vi "oef12.vi"() -> ()   [LabVIEW 2021]
panel:
  out "array sum":dbl
  out "result":dbl[][](array[numeric])
  in  "stop":bool
  out "kernel-sum":dbl[][](array[numeric])
  out "result":dbl
  out "inputElement":i8
  out "kernelElement":dbl
  out "rowKernel":i8[](array[numeric])
  out "rowInput":i8[](array[numeric])
  in  "kernel":dbl[][](array[numeric])
  out "Array":i8[][](array[numeric])
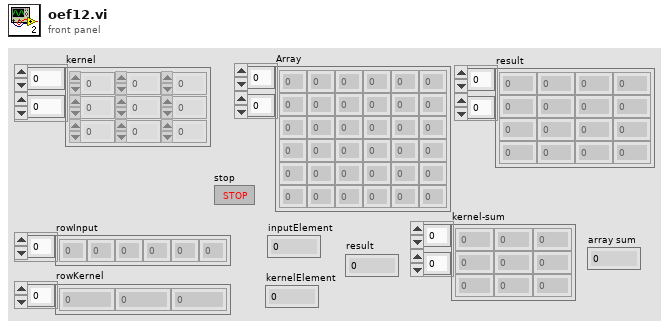
[diagram p1: front panel]
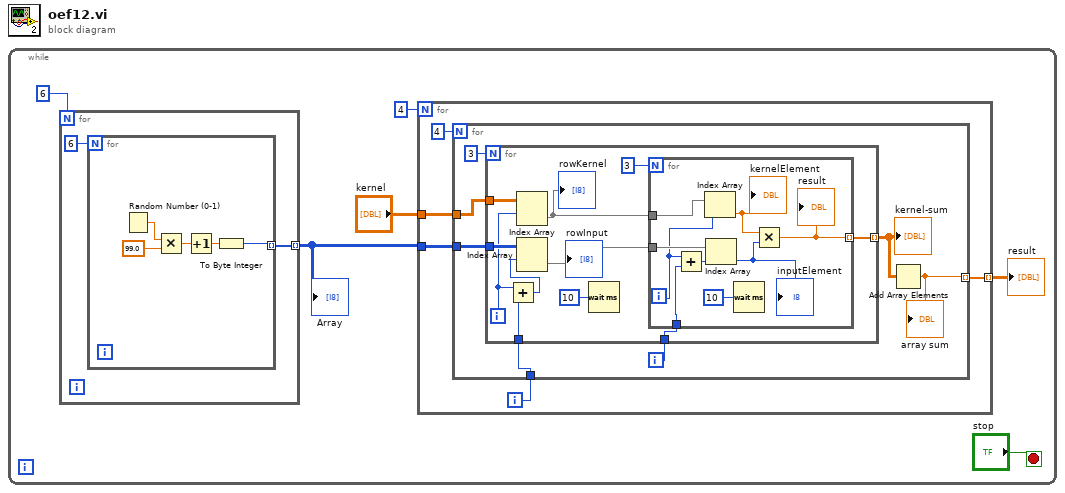
[diagram p0: block diagram]
diagram:
  n1 = while {
    stop <- "stop" stop-if-true
    n2 = for {
      N: 6 -> [_]
      tunnel: [w39] -> w6 mode=indexing
      n3 = for {
        N: 6 -> [_]
        tunnel: [w41] -> w39 mode=indexing
        n4 = Random Number (0-1)() -> (number: 0 to 1=w44:dbl)
        n5 = Multiply(x=w44, y=99.0) -> (x*y=w45:dbl)
        n6 = Increment(x=w45) -> (x+1=w42:dbl)
        n7 = To Byte Integer(number=w42) -> (8bit integer=w41:i8)
      }
    }
    "Array" <- w6
    n8 = for {
      N: 4 -> [_]
      tunnel: w6 -> [w11]
      tunnel: "kernel" -> [w10]
      tunnel: [w7] -> w1 mode=indexing
      i -> [w8]
      n9 = for {
        N: 4 -> [_]
        tunnel: w11 -> [w18]
        tunnel: w10 -> [w17]
        tunnel: w8 -> [w14]
        tunnel: [w12] -> w7 mode=indexing
        i -> [w15]
        n10 = for {
          N: 3 -> [_]
          tunnel: w18 -> [w28]
          tunnel: w17 -> [w25]
          tunnel: w15 -> [w23]
          tunnel: w14 -> [w21]
          tunnel: [w20] -> w13 mode=indexing
          i -> [w22]
          n11 = Add(x=w22, y=w21) -> (x+y=w19:i32)
          n12 = Index Array(array=w25, index (row)=w22) -> (element=w24:dbl[])  [unwired: 1 in]
          "rowKernel" <- w24
          n13 = Index Array(array=w28, index (row)=w19) -> (element=w27:i8[])  [unwired: 1 in]
          "rowInput" <- w27
          n14 = Wait (ms)(milliseconds to wait=u32 10) -> ()  [unwired: 1 out]
          n15 = for {
            N: 3 -> [_]
            tunnel: w27 -> [w36]
            tunnel: w24 -> [w34]
            tunnel: w23 -> [w31]
            tunnel: [w30] -> w20 mode=indexing
            i -> [w32]
            n16 = Add(x=w32, y=w31) -> (x+y=w33:i32)
            n17 = Index Array(array=w34, index=w32) -> (element=w35:dbl)
            "kernelElement" <- w35
            n18 = Index Array(array=w36, index=w33) -> (element=w37:i8)
            "inputElement" <- w37
            n19 = Wait (ms)(milliseconds to wait=u32 10) -> ()  [unwired: 1 out]
            n20 = Multiply(x=w35, y=w37) -> (x*y=w30:dbl)
            "result" <- w30
          }
        }
        "kernel-sum" <- w13
        n21 = Add Array Elements(numeric array=w13) -> (sum=w12:dbl)
        "array sum" <- w12
      }
    }
    "result" <- w1
  }
